vi "Clear Parent.vi"(8 "error in (no error)":errorcluster, 11 "NodeRef In":refnum<data-value>) -> (0 "error out":errorcluster, 3 "NodeRef":refnum<data-value>)   [LabVIEW 2020, in "PicoG-ParserLexer.lvlib" / "Node.lvclass"]
uses:
  Node.lvclass
panel:
  out "Parent":refnum<data-value>
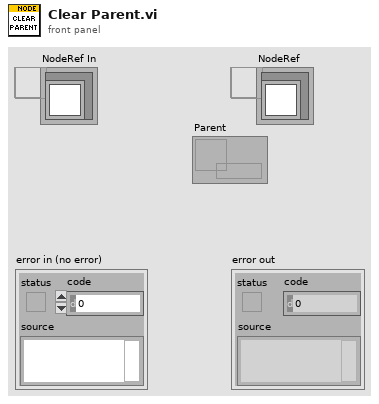
[diagram p1: front panel]
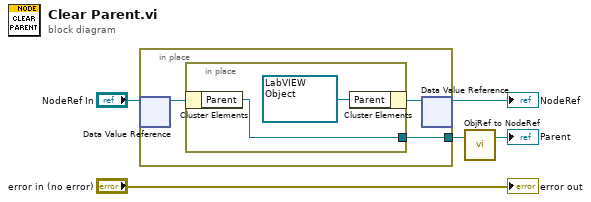
[diagram p0: block diagram]
diagram:
  n1 = in-place {
    in-place-border: [w6] -> w2
    n2 = in-place-dvr #1("NodeRef In") -> (w8:refnum<class "Node.lvclass">)  [unwired: 1 out]
    n3 = in-place {
      in-place-border: [w9] -> w6
      n4 = in-place-cluster #2(w8) -> ("Parent"=w9:refnum<data-value>)
      n5 = in-place-cluster #2("Parent"=refnum<data-value> refnum) -> (w7:refnum<class "Node.lvclass">)
    }
    n6 = in-place-dvr #1(w7) -> (→"NodeRef":refnum<data-value>)  [unwired: 1 out]
  }
  n7 = call "ObjRef to NodeRef.vi"("ObjectRef"=w2) -> ("NodeRef"=→"Parent":refnum<data-value>)  [unwired: 2 in]
  "error out" <- "error in (no error)"
